vi "CamerasBegin.vi"   [LabVIEW 2017]
uses:
  <vilib>/Rock Robotics/WPI/Camera/WPI_CameraWhite Balance Values.ctl
  <vilib>/Rock Robotics/WPI/Camera/WPI_CameraFrameRate.ctl
  <vilib>/Rock Robotics/WPI/Camera/WPI_CameraExposure Values.ctl
  Robot Global Data.vi
  <vilib>/Rock Robotics/Network Tables/NT Write String.vi
types:
  T1 = typedef "WPI_CameraFrameRate.ctl" = u32
  T2 = typedef "WPI_CameraWhite Balance Values.ctl" = enum16{"Auto", "Fixed indoor", "Fixed outdoor 1", "Fixed outdoor 2", "Fixed fluorescent 1", "Fixed fluorescent 2", "Hold current", "Custom"}
  T3 = typedef "WPI_CameraExposure Values.ctl" = enum16{"Auto", "Flicker-free 50 Hz", "Flicker-free 60 Hz", "Hold current", "Custom"}
  T4 = typedef "WPI_CameraDevRef.ctl" = cluster{"Camera Address":string, "CameraStatus":errorcluster}
  T5 = typedef "WPI_CameraImageSize.ctl" = enum16{"640x480", "320x240", "160x120", "Custom"}
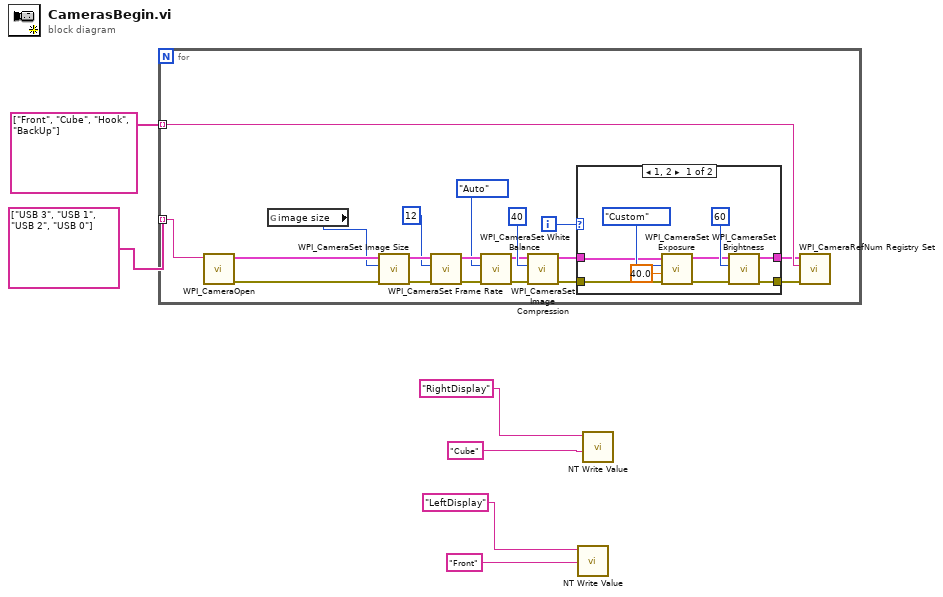
[diagram p0: block diagram]
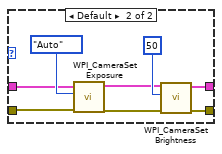
[diagram p2: hidden frame]
diagram:
  n1 = for {
    tunnel: string[] ["Front", "Cube", "Hook", "BackUp"] ("refnum name") -> [w25] mode=indexing
    tunnel: string[] ["USB 3", "USB 1", "USB 2", "USB 0"] ("format string") -> [w20] mode=indexing
    i -> [w9]
    n2 = call <vilib>:"WPI_CameraOpen.vi"("Camera Address"=w20) -> ("error out"=w23:errorcluster, "CameraDevRef"=w24:T4)  [unwired: 1 in, 8 out]
    n3 = global read "Robot Global Data.vi" "image size"() -> (w10:T5)
    n4 = call <vilib>:"WPI_CameraSet Image Size.vi"("error in (no error)"=w23, "Image Size"=w10, "CameraDevRef"=w24) -> ("error out"=w15:errorcluster, "CameraDevRef Out"=w16:T4)  [unwired: 1 in, 6 out]
    n5 = call <vilib>:"WPI_CameraSet Frame Rate.vi"("error in (no error)"=w15, "Frame Rate (fps)"=T1 12, "CameraDevRef"=w16) -> ("error out"=w14:errorcluster, "CameraDevRef Out"=w17:T4)  [unwired: 7 out]
    n6 = call <vilib>:"WPI_CameraSet White Balance.vi"("error in (no error)"=w14, "White Balance"=WPI_CameraWhite_Balance_Values."Auto", "CameraDevRef"=w17) -> ("error out"=w7:errorcluster, "CameraDevRef Out"=w8:T4)  [unwired: 1 in, 6 out]
    n7 = call <vilib>:"WPI_CameraSet Image Compression.vi"("error in (no error)"=w7, "Compression"=40, "CameraDevRef"=w8) -> ("error out"=w13:errorcluster, "CameraDevRef Out"=w18:T4)  [unwired: 7 out]
    n8 = case shown="1, 2" w9 {
      tunnel: [w34 w42] -> w22
      tunnel: [w33 w41] -> w21
      tunnel: w18 -> [w30 w38]
      tunnel: w13 -> [w29 w35]
      frame 1, 2 {
        n9 = call <vilib>:"WPI_CameraSet Exposure.vi"("error in (no error)"=w29, "Exposure (%)"=40.0, "Exposure"=WPI_CameraExposure_Values."Custom", "CameraDevRef"=w30) -> ("error out"=w28:errorcluster, "CameraDevRef Out"=w27:T4)  [unwired: 6 out]
        n10 = call <vilib>:"WPI_CameraSet Brightness.vi"("error in (no error)"=w28, "Brightness"=60, "CameraDevRef"=w27) -> ("error out"=w33:errorcluster, "CameraDevRef Out"=w34:T4)  [unwired: 1 in, 6 out]
      }
      frame Default {
        n11 = call <vilib>:"WPI_CameraSet Exposure.vi"("error in (no error)"=w35, "Exposure"=WPI_CameraExposure_Values."Auto", "CameraDevRef"=w38) -> ("error out"=w36:errorcluster, "CameraDevRef Out"=w37:T4)  [unwired: 1 in, 6 out]
        n12 = call <vilib>:"WPI_CameraSet Brightness.vi"("error in (no error)"=w36, "Brightness"=50, "CameraDevRef"=w37) -> ("error out"=w41:errorcluster, "CameraDevRef Out"=w42:T4)  [unwired: 1 in, 6 out]
      }
    }
    n13 = call <vilib>:"WPI_CameraRefNum Registry Set.vi"("error in (no error)"=w21, "refnum name"=w25, "CameraDevRef"=w22) -> ()  [unwired: 1 in, 8 out]
  }
  n14 = call-poly <vilib>:"NT Write Value.vi"("String"="Front" ("refnum name"), "Name"="LeftDisplay") -> ()  [unwired: 9 in, 1 out]
  n15 = call-poly <vilib>:"NT Write Value.vi"("String"="Cube" ("refnum name"), "Name"="RightDisplay") -> ()  [unwired: 9 in, 1 out]
